vi "LD2018_ブロック崩し_Main.vi"() -> ()   [LabVIEW 2016]
uses:
  <vilib>/Utility/inputDevices.llb/keyboardAcquire.vi
  <vilib>/Utility/inputDevices.llb/closeKeyboard.vi
panel:
  out "Stage":i32
  out "残機":i32
  out "Combo":i32
  out "Combo":bool
  out "SCORE":i32
  out "BL 0":bool
  out "BL 1":bool
  out "BL 2":bool
  out "BL 3":bool
  out "BL 4":bool
  out "BL 5":bool
  out "BL 6":bool
  out "BL 7":bool
  out "BL 8":bool
  out "BL 9":bool
  out "BL 10":bool
  out "BL 11":bool
  out "BL 12":bool
  out "BL 13":bool
  out "BL 14":bool
  out "BL 15":bool
  out "BL 16":bool
  out "BL 17":bool
  out "BL 18":bool
  out "BL 19":bool
  out "BL 20":bool
  out "BL 21":bool
  out "BL 22":bool
  out "BL 23":bool
  out "BL 24":bool
  out "BL 25":bool
  out "BL 26":bool
  out "BL 27":bool
  out "BL 28":bool
  out "BL 29":bool
  out "BL 30":bool
  out "BL 31":bool
  out "BL 32":bool
  out "BL 33":bool
  out "BL 34":bool
  out "BL 35":bool
  out "BL 36":bool
  out "BL 37":bool
  out "BL 38":bool
  out "BL 39":bool
  out "BL 40":bool
  out "BL 41":bool
  out "BL 42":bool
  out "BL 43":bool
  out "BL 44":bool
  out "BL 45":bool
  out "BL 46":bool
  out "BL 47":bool
  out "BL 48":bool
  out "BL 49":bool
  out "BL 50":bool
  out "BL 51":bool
  out "BL 52":bool
  out "BL 53":bool
  out "BL 54":bool
  out "BL 55":bool
  out "BL 56":bool
  out "BL 57":bool
  out "BL 58":bool
  out "BL 59":bool
  out "BL 60":bool
  out "BL 61":bool
  out "BL 62":bool
  out "BL 63":bool
  out "BL 64":bool
  out "BL 65":bool
  out "BL 66":bool
  out "BL 67":bool
  out "BL 68":bool
  out "BL 69":bool
  out "BL 70":bool
  out "BL 71":bool
  out "BL 72":bool
  out "BL 73":bool
  out "BL 74":bool
  out "BL 75":bool
  out "BL 76":bool
  out "BL 77":bool
  out "BL 78":bool
  out "BL 79":bool
  out "BL 80":bool
  out "BL 81":bool
  out "BL 82":bool
  out "BL 83":bool
  out "BL 84":bool
  out "BL 85":bool
  out "BL 86":bool
  out "BL 87":bool
  out "BL 88":bool
  out "BL 89":bool
  out "BL 90":bool
  out "BL 91":bool
  out "BL 92":bool
  out "BL 93":bool
  out "BL 94":bool
  out "BL 95":bool
  out "BL 96":bool
  out "BL 97":bool
  out "BL 98":bool
  out "BL 99":bool
  out "BL 100":bool
  out "BL 110":bool
  out "BL 120":bool
  out "BL 130":bool
  out "BL 140":bool
  out "BL 101":bool
  out "BL 111":bool
  out "BL 121":bool
  out "BL 131":bool
  out "BL 141":bool
  out "BL 102":bool
  out "BL 112":bool
  out "BL 122":bool
  out "BL 132":bool
  out "BL 142":bool
  out "BL 103":bool
  out "BL 113":bool
  out "BL 123":bool
  out "BL 133":bool
  out "BL 143":bool
  out "BL 104":bool
  out "BL 114":bool
  out "BL 124":bool
  out "BL 134":bool
  out "BL 144":bool
  out "BL 105":bool
  out "BL 115":bool
  out "BL 125":bool
  out "BL 135":bool
  out "BL 145":bool
  out "BL 106":bool
  out "BL 116":bool
  out "BL 126":bool
  out "BL 136":bool
  out "BL 146":bool
  out "BL 107":bool
  out "BL 117":bool
  out "BL 127":bool
  out "BL 137":bool
  out "BL 147":bool
  out "BL 108":bool
  out "BL 118":bool
  out "BL 128":bool
  out "BL 138":bool
  out "BL 148":bool
  out "BL 109":bool
  out "BL 119":bool
  out "BL 129":bool
  out "BL 139":bool
  out "BL 149":bool
  out "x - y":u32
  in  "rect":T1={"left"=175, "top"=550, "right"=224, "bottom"=565} caption="長方形"
  out "Scrn-PADDLE":picture
  out "Scrn-BALL":picture
  # "BGカラーを黒(#000000)にすると\n処理速度が上がる？"
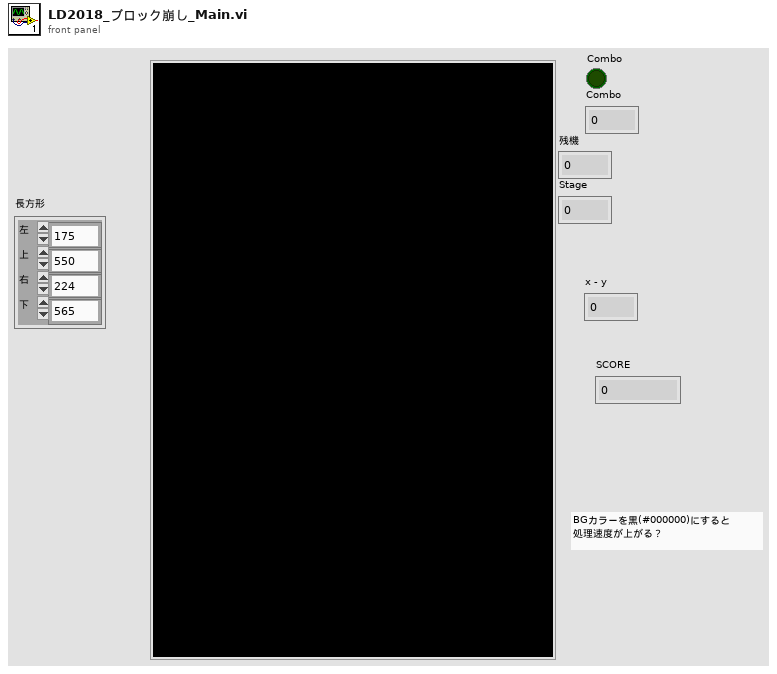
[diagram p1: front panel]
types:
  T1 = cluster{"left":i16, "top":i16, "right":i16, "bottom":i16}
  T2 = cluster{"left":dbl, "top":dbl, "right":dbl, "bottom":dbl}
  T3 = enum16{"0", "1", "2", "3", "4", "5", "6", "7", "8", "9", "A", "B", "C", "D", "E", "F", "G", "H", "I", "J", "K", "L", "M", "N", "O", "P", "Q", "R", "S", "T", "U", "V", "W", "X", "Y", "Z", "F1", "F2", "F3", "F4", "F5", "F6", "F7", "F8", "F9", "F10", "F11", "F12", "F13", "F14", "F15", "ADD", "BACK", "BACKSLASH", "CAPITAL", "COMMA", "DECIMAL", "DELETE", "DIVIDE", "DOWN", "END", "EQUALS", "ESCAPE", "GRAVE (`)", "HOME", "INSERT", "LBRACKET", "LCONTROL", "LEFT", "L ALT", "LSHIFT", "LWIN", "MINUS", "MULTIPLY", "NEXT", "NUMLOCK", "NUMPAD_0", "NUMPAD_1", "NUMPAD_2", "NUMPAD_3", "NUMPAD_4", "NUMPAD_5", "NUMPAD_6", "NUMPAD_7", "NUMPAD_8", "NUMPAD_9", "PAUSE", "PERIOD", "PRIOR (PG UP)", "RBRACKET", "RCONTROL", "RETURN", "RIGHT", "R ALT", "RSHIFT", "RWIN", "SCROLL", "SEMICOLON", "SLASH", "SPACE", "SUBTRACT", "TAB", "UP", "ENTER (num pad)", "' (quote)"}[]
  T4 = typedef "LVPositionTypeDef.ctl" = cluster{"Left":i32, "Top":i32}
  T5 = enum16{"0", "1", "2", "3", "4", "5", "6", "7", "8", "9", "A", "B", "C", "D", "E", "F", "G", "H", "I", "J", "K", "L", "M", "N", "O", "P", "Q", "R", "S", "T", "U", "V", "W", "X", "Y", "Z", "F1", "F2", "F3", "F4", "F5", "F6", "F7", "F8", "F9", "F10", "F11", "F12", "F13", "F14", "F15", "ADD", "BACK", "BACKSLASH", "CAPITAL", "COMMA", "DECIMAL", "DELETE", "DIVIDE", "DOWN", "END", "EQUALS", "ESCAPE", "GRAVE (`)", "HOME", "INSERT", "LBRACKET", "LCONTROL", "LEFT", "L ALT", "LSHIFT", "LWIN", "MINUS", "MULTIPLY", "NEXT", "NUMLOCK", "NUMPAD_0", "NUMPAD_1", "NUMPAD_2", "NUMPAD_3", "NUMPAD_4", "NUMPAD_5", "NUMPAD_6", "NUMPAD_7", "NUMPAD_8", "NUMPAD_9", "PAUSE", "PERIOD", "PRIOR (PG UP)", "RBRACKET", "RCONTROL", "RETURN", "RIGHT", "R ALT", "RSHIFT", "RWIN", "SCROLL", "SEMICOLON", "SLASH", "SPACE", "SUBTRACT", "TAB", "UP", "ENTER (num pad)", "' (quote)"}
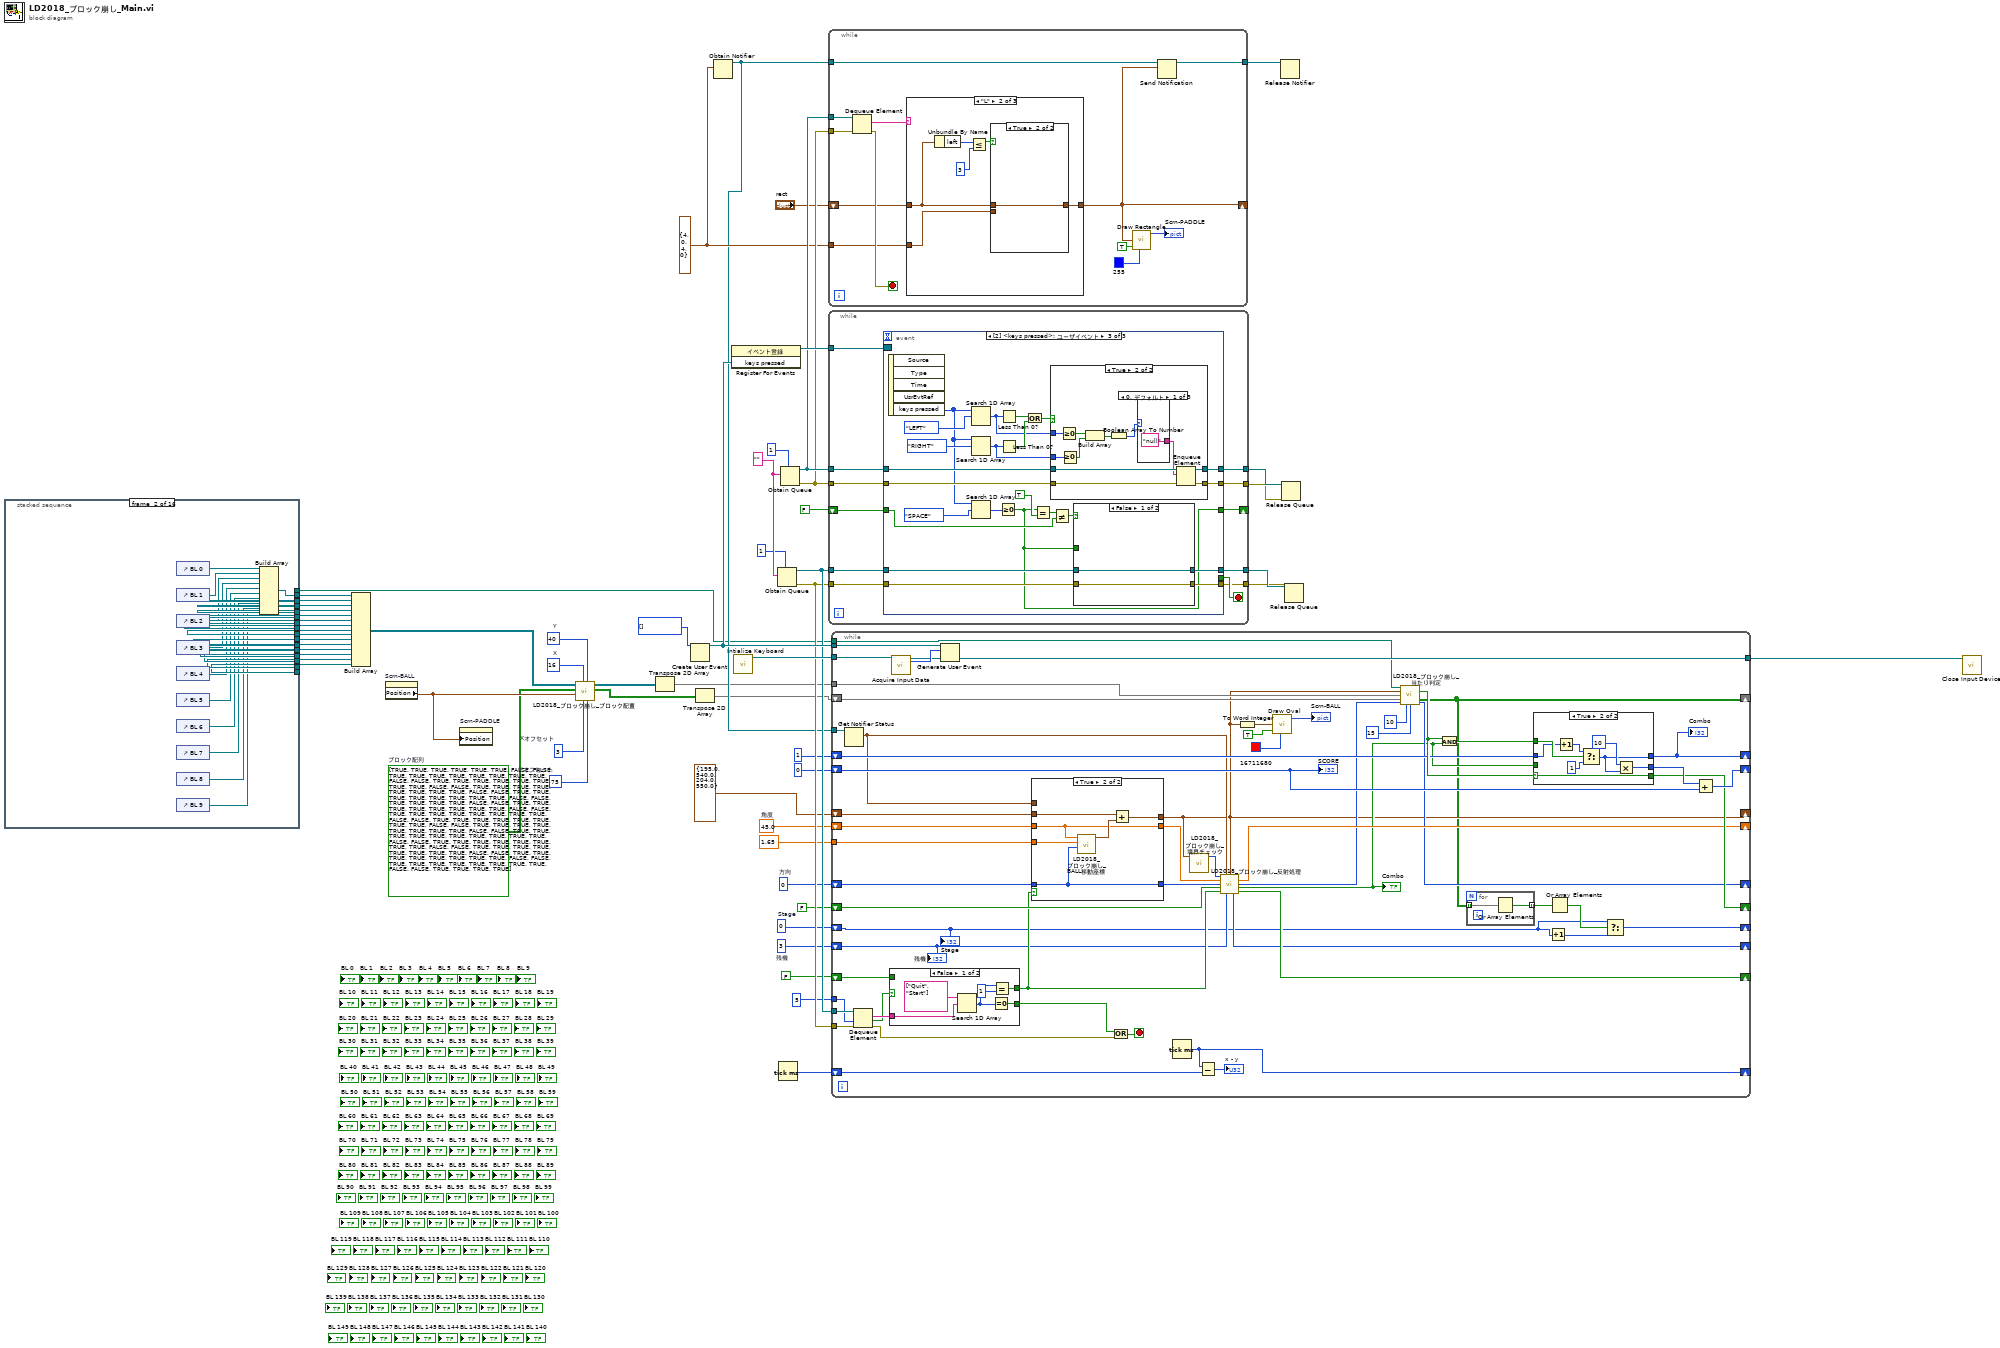
[diagram p0: block diagram]
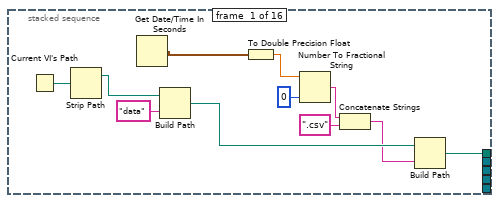
[diagram p2: hidden frame]
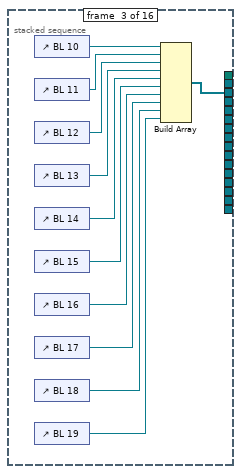
[diagram p3: hidden frame]
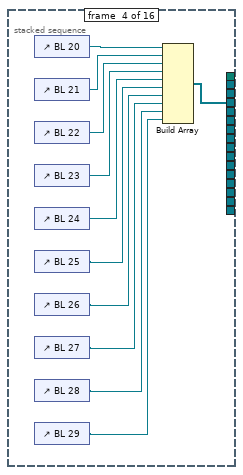
[diagram p4: hidden frame]
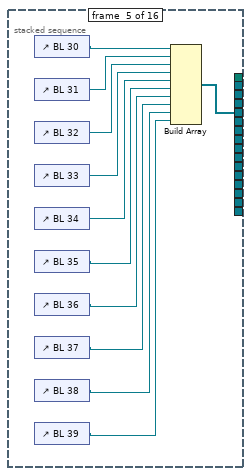
[diagram p5: hidden frame]
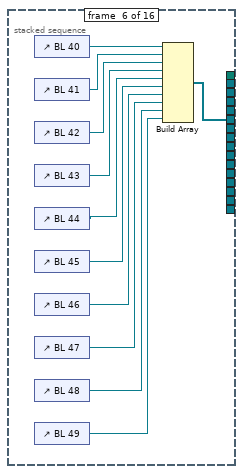
[diagram p6: hidden frame]
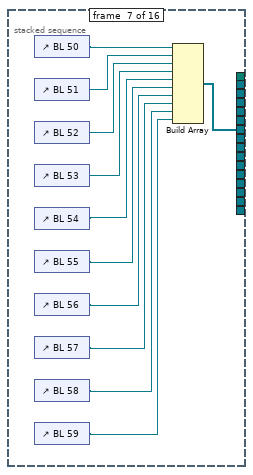
[diagram p7: hidden frame]
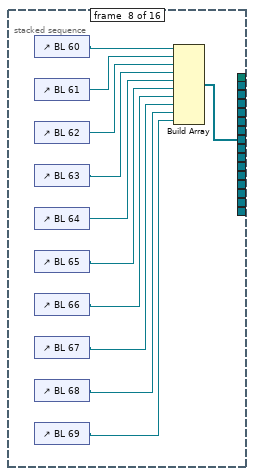
[diagram p8: hidden frame]
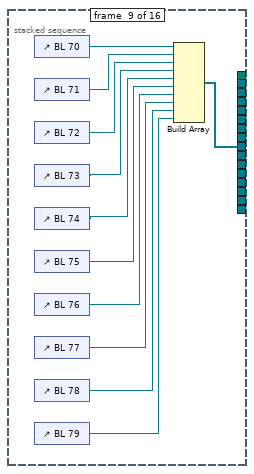
[diagram p9: hidden frame]
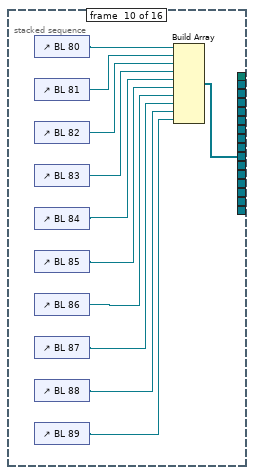
[diagram p10: hidden frame]
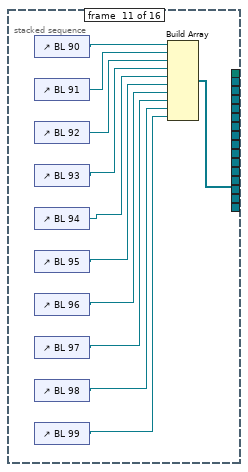
[diagram p11: hidden frame]
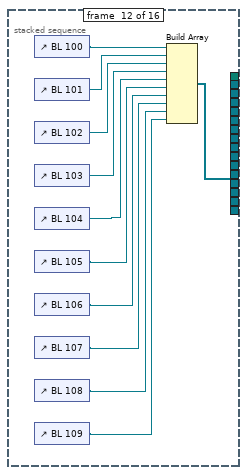
[diagram p12: hidden frame]
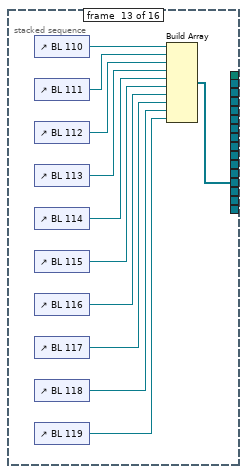
[diagram p13: hidden frame]
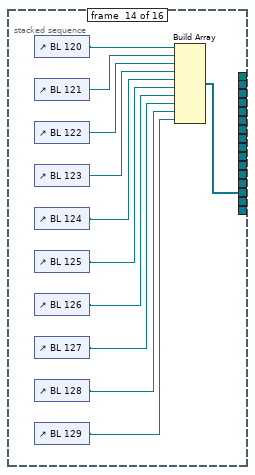
[diagram p14: hidden frame]
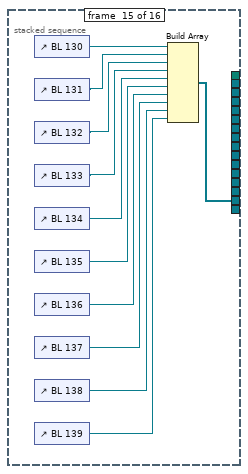
[diagram p15: hidden frame]
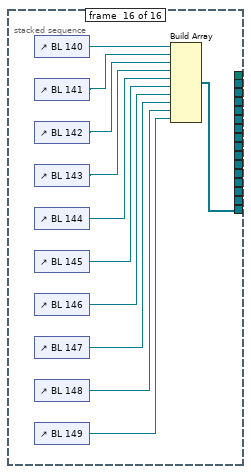
[diagram p16: hidden frame]
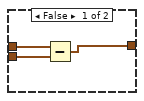
[diagram p18: hidden frame]
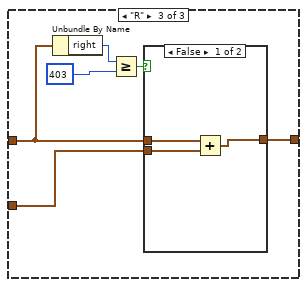
[diagram p19: hidden frame]
diagram:
  w1 = 3  # 残機
  w2 = 0  # Stage
  w8 = 75  # Yオフセット
  w9 = 3  # Xオフセット
  w10 = 40  # Y
  w11 = 16  # X
  w5 = bool[][] [[TRUE, TRUE, TRUE, TRUE, TRUE, TRUE, FALSE, FALSE, TRUE, TRUE], [TRUE, TRUE, TRUE, TRUE, TRUE, TRUE, FALSE, FALSE, TRUE, TRUE], [TRUE, TRUE, TRUE, TRUE, TRUE, TRUE, FALSE, FALSE, TRUE, TRUE], [TRUE, TRUE, TRUE, TRUE, TRUE, TRUE, FALSE, FALSE, TRUE, TRUE], [TRUE, TRUE, TRUE, TRUE, TRUE, TRUE, FALSE, FALSE, TRUE, TRUE], [TRUE, TRUE, FALSE, FALSE, TRUE, TRUE, TRUE, TRUE, TRUE, TRUE], [TRUE, TRUE, FALSE, FALSE, TRUE, TRUE, TRUE, TRUE, TRUE, TRUE], [TRUE, TRUE, FALSE, FALSE, TRUE, TRUE, TRUE, TRUE, TRUE, TRUE], [TRUE, TRUE, FALSE, FALSE, TRUE, TRUE, TRUE, TRUE, TRUE, TRUE], [TRUE, TRUE, FALSE, FALSE, TRUE, TRUE, TRUE, TRUE, TRUE, TRUE], [TRUE, TRUE, TRUE, TRUE, FALSE, FALSE, TRUE, TRUE, TRUE, TRUE], [TRUE, TRUE, TRUE, TRUE, FALSE, FALSE, TRUE, TRUE, TRUE, TRUE], [TRUE, TRUE, TRUE, TRUE, FALSE, FALSE, TRUE, TRUE, TRUE, TRUE], [TRUE, TRUE, TRUE, TRUE, FALSE, FALSE, TRUE, TRUE, TRUE, TRUE], [TRUE, TRUE, TRUE, TRUE, FALSE, FALSE, TRUE, TRUE, TRUE, TRUE]]  # ブロック配列
  w44 = 0  # 方向
  w45 = 45.0  # 角度
  w33 = T1 {"left"=4, "top"=0, "right"=4, "bottom"=0} ("rect")
  w16 = ""
  w59 = T3 [] items=["0", "1", "2", "3", "4", "5", "6", "7", "8", "9", "A", "B", "C", "D", "E", "F", "G", "H", "I", "J", "K", "L", "M", "N", "O", "P", "Q", "R", "S", "T", "U", "V", "W", "X", "Y", "Z", "F1", "F2", "F3", "F4", "F5", "F6", "F7", "F8", "F9", "F10", "F11", "F12", "F13", "F14", "F15", "ADD", "BACK", "BACKSLASH", "CAPITAL", "COMMA", "DECIMAL", "DELETE", "DIVIDE", "DOWN", "END", "EQUALS", "ESCAPE", "GRAVE (`)", "HOME", "INSERT", "LBRACKET", "LCONTROL", "LEFT", "L ALT", "LSHIFT", "LWIN", "MINUS", "MULTIPLY", "NEXT", "NUMLOCK", "NUMPAD_0", "NUMPAD_1", "NUMPAD_2", "NUMPAD_3", "NUMPAD_4", "NUMPAD_5", "NUMPAD_6", "NUMPAD_7", "NUMPAD_8", "NUMPAD_9", "PAUSE", "PERIOD", "PRIOR (PG UP)", "RBRACKET", "RCONTROL", "RETURN", "RIGHT", "R ALT", "RSHIFT", "RWIN", "SCROLL", "SEMICOLON", "SLASH", "SPACE", "SUBTRACT", "TAB", "UP", "ENTER (num pad)", "' (quote)"] ("keys pressed")
  n1 = stacked-sequence {
    tunnel: [_ w72 _ _ _ _ _ _ _ _ _ _ _ _ _ _] -> w43
    tunnel: [_ _ w83 _ _ _ _ _ _ _ _ _ _ _ _ _] -> w42
    tunnel: [_ _ _ w104 _ _ _ _ _ _ _ _ _ _ _ _] -> w41
    tunnel: [_ _ _ _ w115 _ _ _ _ _ _ _ _ _ _ _] -> w40
    tunnel: [_ _ _ _ _ w126 _ _ _ _ _ _ _ _ _ _] -> w39
    tunnel: [_ _ _ _ _ _ w137 _ _ _ _ _ _ _ _ _] -> w38
    tunnel: [_ _ _ _ _ _ _ w148 _ _ _ _ _ _ _ _] -> w37
    tunnel: [_ _ _ _ _ _ _ _ w159 _ _ _ _ _ _ _] -> w36
    tunnel: [_ _ _ _ _ _ _ _ _ w170 _ _ _ _ _ _] -> w35
    tunnel: [_ _ _ _ _ _ _ _ _ _ w181 _ _ _ _ _] -> w34
    tunnel: [_ _ _ _ _ _ _ _ _ _ _ w182 _ _ _ _] -> w27
    tunnel: [_ _ _ _ _ _ _ _ _ _ _ _ w193 _ _ _] -> w26
    tunnel: [_ _ _ _ _ _ _ _ _ _ _ _ _ w205 _ _] -> w25
    tunnel: [_ _ _ _ _ _ _ _ _ _ _ _ _ _ w215 _] -> w24
    tunnel: [_ _ _ _ _ _ _ _ _ _ _ _ _ _ _ w226] -> w23
    tunnel: [w62 _ _ _ _ _ _ _ _ _ _ _ _ _ _ _] -> w20
    frame #0 {
      n2 = Current VI's Path() -> (path=w69:path)
      n3 = Strip Path(path=w69) -> (stripped path=w70:path)  [unwired: 1 out]
      n4 = Get Date/Time In Seconds() -> (seconds since 1Jan1904=w61:timestamp)
      n5 = Build Path(base path=w70, name or relative path="data" ("名前または相対パス")) -> (appended path=w64:path)
      n6 = To Double Precision Float(number=w61) -> (double precision float=w68:dbl)
      n7 = Number To Fractional String(number=w68, precision (6)=i16 0 ("精度（6）")) -> (F-format string=w66:string)  [unwired: 2 in]
      n8 = Concatenate Strings(w66, ".csv" ("文字列")) -> (w63:string)
      n9 = Build Path(base path=w64, name or relative path=w63) -> (appended path=w62:path)
    }
    frame #1 {
      n10 = control-ref of="BL 0"() -> (w73:refnum<vi>)
      n11 = control-ref of="BL 1"() -> (w74:refnum<vi>)
      n12 = control-ref of="BL 2"() -> (w75:refnum<vi>)
      n13 = control-ref of="BL 3"() -> (w76:refnum<vi>)
      n14 = control-ref of="BL 4"() -> (w77:refnum<vi>)
      n15 = control-ref of="BL 5"() -> (w78:refnum<vi>)
      n16 = control-ref of="BL 6"() -> (w79:refnum<vi>)
      n17 = control-ref of="BL 7"() -> (w80:refnum<vi>)
      n18 = control-ref of="BL 8"() -> (w81:refnum<vi>)
      n19 = control-ref of="BL 9"() -> (w82:refnum<vi>)
      n20 = Build Array(w73, w74, w75, w76, w77, w78, w79, w80, w81, w82) -> (w72:refnum<vi>[])
    }
    frame #2 {
      n21 = control-ref of="BL 10"() -> (w93:refnum<vi>)
      n22 = control-ref of="BL 11"() -> (w92:refnum<vi>)
      n23 = control-ref of="BL 12"() -> (w91:refnum<vi>)
      n24 = control-ref of="BL 13"() -> (w90:refnum<vi>)
      n25 = control-ref of="BL 14"() -> (w89:refnum<vi>)
      n26 = control-ref of="BL 15"() -> (w88:refnum<vi>)
      n27 = control-ref of="BL 16"() -> (w87:refnum<vi>)
      n28 = control-ref of="BL 17"() -> (w86:refnum<vi>)
      n29 = control-ref of="BL 18"() -> (w85:refnum<vi>)
      n30 = control-ref of="BL 19"() -> (w84:refnum<vi>)
      n31 = Build Array(w93, w92, w91, w90, w89, w88, w87, w86, w85, w84) -> (w83:refnum<vi>[])
    }
    frame #3 {
      n32 = control-ref of="BL 20"() -> (w103:refnum<vi>)
      n33 = control-ref of="BL 21"() -> (w102:refnum<vi>)
      n34 = control-ref of="BL 22"() -> (w101:refnum<vi>)
      n35 = control-ref of="BL 23"() -> (w100:refnum<vi>)
      n36 = control-ref of="BL 24"() -> (w99:refnum<vi>)
      n37 = control-ref of="BL 25"() -> (w98:refnum<vi>)
      n38 = control-ref of="BL 26"() -> (w97:refnum<vi>)
      n39 = control-ref of="BL 27"() -> (w96:refnum<vi>)
      n40 = control-ref of="BL 28"() -> (w95:refnum<vi>)
      n41 = control-ref of="BL 29"() -> (w94:refnum<vi>)
      n42 = Build Array(w103, w102, w101, w100, w99, w98, w97, w96, w95, w94) -> (w104:refnum<vi>[])
    }
    frame #4 {
      n43 = control-ref of="BL 30"() -> (w114:refnum<vi>)
      n44 = control-ref of="BL 31"() -> (w113:refnum<vi>)
      n45 = control-ref of="BL 32"() -> (w112:refnum<vi>)
      n46 = control-ref of="BL 33"() -> (w111:refnum<vi>)
      n47 = control-ref of="BL 34"() -> (w110:refnum<vi>)
      n48 = control-ref of="BL 35"() -> (w109:refnum<vi>)
      n49 = control-ref of="BL 36"() -> (w108:refnum<vi>)
      n50 = control-ref of="BL 37"() -> (w107:refnum<vi>)
      n51 = control-ref of="BL 38"() -> (w106:refnum<vi>)
      n52 = control-ref of="BL 39"() -> (w105:refnum<vi>)
      n53 = Build Array(w114, w113, w112, w111, w110, w109, w108, w107, w106, w105) -> (w115:refnum<vi>[])
    }
    frame #5 {
      n54 = control-ref of="BL 40"() -> (w125:refnum<vi>)
      n55 = control-ref of="BL 41"() -> (w124:refnum<vi>)
      n56 = control-ref of="BL 42"() -> (w123:refnum<vi>)
      n57 = control-ref of="BL 43"() -> (w122:refnum<vi>)
      n58 = control-ref of="BL 44"() -> (w121:refnum<vi>)
      n59 = control-ref of="BL 45"() -> (w120:refnum<vi>)
      n60 = control-ref of="BL 46"() -> (w119:refnum<vi>)
      n61 = control-ref of="BL 47"() -> (w118:refnum<vi>)
      n62 = control-ref of="BL 48"() -> (w117:refnum<vi>)
      n63 = control-ref of="BL 49"() -> (w116:refnum<vi>)
      n64 = Build Array(w125, w124, w123, w122, w121, w120, w119, w118, w117, w116) -> (w126:refnum<vi>[])
    }
    frame #6 {
      n65 = control-ref of="BL 50"() -> (w136:refnum<vi>)
      n66 = control-ref of="BL 51"() -> (w135:refnum<vi>)
      n67 = control-ref of="BL 52"() -> (w134:refnum<vi>)
      n68 = control-ref of="BL 53"() -> (w133:refnum<vi>)
      n69 = control-ref of="BL 54"() -> (w132:refnum<vi>)
      n70 = control-ref of="BL 55"() -> (w131:refnum<vi>)
      n71 = control-ref of="BL 56"() -> (w130:refnum<vi>)
      n72 = control-ref of="BL 57"() -> (w129:refnum<vi>)
      n73 = control-ref of="BL 58"() -> (w128:refnum<vi>)
      n74 = control-ref of="BL 59"() -> (w127:refnum<vi>)
      n75 = Build Array(w136, w135, w134, w133, w132, w131, w130, w129, w128, w127) -> (w137:refnum<vi>[])
    }
    frame #7 {
      n76 = control-ref of="BL 60"() -> (w147:refnum<vi>)
      n77 = control-ref of="BL 61"() -> (w146:refnum<vi>)
      n78 = control-ref of="BL 62"() -> (w145:refnum<vi>)
      n79 = control-ref of="BL 63"() -> (w144:refnum<vi>)
      n80 = control-ref of="BL 64"() -> (w143:refnum<vi>)
      n81 = control-ref of="BL 65"() -> (w142:refnum<vi>)
      n82 = control-ref of="BL 66"() -> (w141:refnum<vi>)
      n83 = control-ref of="BL 67"() -> (w140:refnum<vi>)
      n84 = control-ref of="BL 68"() -> (w139:refnum<vi>)
      n85 = control-ref of="BL 69"() -> (w138:refnum<vi>)
      n86 = Build Array(w147, w146, w145, w144, w143, w142, w141, w140, w139, w138) -> (w148:refnum<vi>[])
    }
    frame #8 {
      n87 = control-ref of="BL 70"() -> (w158:refnum<vi>)
      n88 = control-ref of="BL 71"() -> (w157:refnum<vi>)
      n89 = control-ref of="BL 72"() -> (w156:refnum<vi>)
      n90 = control-ref of="BL 73"() -> (w155:refnum<vi>)
      n91 = control-ref of="BL 74"() -> (w154:refnum<vi>)
      n92 = control-ref of="BL 75"() -> (w153:refnum<vi>)
      n93 = control-ref of="BL 76"() -> (w152:refnum<vi>)
      n94 = control-ref of="BL 77"() -> (w151:refnum<vi>)
      n95 = control-ref of="BL 78"() -> (w150:refnum<vi>)
      n96 = control-ref of="BL 79"() -> (w149:refnum<vi>)
      n97 = Build Array(w158, w157, w156, w155, w154, w153, w152, w151, w150, w149) -> (w159:refnum<vi>[])
    }
    frame #9 {
      n98 = control-ref of="BL 80"() -> (w169:refnum<vi>)
      n99 = control-ref of="BL 81"() -> (w168:refnum<vi>)
      n100 = control-ref of="BL 82"() -> (w167:refnum<vi>)
      n101 = control-ref of="BL 83"() -> (w166:refnum<vi>)
      n102 = control-ref of="BL 84"() -> (w165:refnum<vi>)
      n103 = control-ref of="BL 85"() -> (w164:refnum<vi>)
      n104 = control-ref of="BL 86"() -> (w163:refnum<vi>)
      n105 = control-ref of="BL 87"() -> (w162:refnum<vi>)
      n106 = control-ref of="BL 88"() -> (w161:refnum<vi>)
      n107 = control-ref of="BL 89"() -> (w160:refnum<vi>)
      n108 = Build Array(w169, w168, w167, w166, w165, w164, w163, w162, w161, w160) -> (w170:refnum<vi>[])
    }
    frame #10 {
      n109 = control-ref of="BL 90"() -> (w180:refnum<vi>)
      n110 = control-ref of="BL 91"() -> (w179:refnum<vi>)
      n111 = control-ref of="BL 92"() -> (w178:refnum<vi>)
      n112 = control-ref of="BL 93"() -> (w177:refnum<vi>)
      n113 = control-ref of="BL 94"() -> (w176:refnum<vi>)
      n114 = control-ref of="BL 95"() -> (w175:refnum<vi>)
      n115 = control-ref of="BL 96"() -> (w174:refnum<vi>)
      n116 = control-ref of="BL 97"() -> (w173:refnum<vi>)
      n117 = control-ref of="BL 98"() -> (w172:refnum<vi>)
      n118 = control-ref of="BL 99"() -> (w171:refnum<vi>)
      n119 = Build Array(w180, w179, w178, w177, w176, w175, w174, w173, w172, w171) -> (w181:refnum<vi>[])
    }
    frame #11 {
      n120 = control-ref of="BL 100"() -> (w192:refnum<vi>)
      n121 = control-ref of="BL 101"() -> (w191:refnum<vi>)
      n122 = control-ref of="BL 102"() -> (w190:refnum<vi>)
      n123 = control-ref of="BL 103"() -> (w189:refnum<vi>)
      n124 = control-ref of="BL 104"() -> (w188:refnum<vi>)
      n125 = control-ref of="BL 105"() -> (w187:refnum<vi>)
      n126 = control-ref of="BL 106"() -> (w186:refnum<vi>)
      n127 = control-ref of="BL 107"() -> (w185:refnum<vi>)
      n128 = control-ref of="BL 108"() -> (w184:refnum<vi>)
      n129 = control-ref of="BL 109"() -> (w183:refnum<vi>)
      n130 = Build Array(w192, w191, w190, w189, w188, w187, w186, w185, w184, w183) -> (w182:refnum<vi>[])
    }
    frame #12 {
      n131 = control-ref of="BL 110"() -> (w203:refnum<vi>)
      n132 = control-ref of="BL 111"() -> (w202:refnum<vi>)
      n133 = control-ref of="BL 112"() -> (w201:refnum<vi>)
      n134 = control-ref of="BL 113"() -> (w200:refnum<vi>)
      n135 = control-ref of="BL 114"() -> (w199:refnum<vi>)
      n136 = control-ref of="BL 115"() -> (w198:refnum<vi>)
      n137 = control-ref of="BL 116"() -> (w197:refnum<vi>)
      n138 = control-ref of="BL 117"() -> (w196:refnum<vi>)
      n139 = control-ref of="BL 118"() -> (w195:refnum<vi>)
      n140 = control-ref of="BL 119"() -> (w194:refnum<vi>)
      n141 = Build Array(w203, w202, w201, w200, w199, w198, w197, w196, w195, w194) -> (w193:refnum<vi>[])
    }
    frame #13 {
      n142 = control-ref of="BL 120"() -> (w214:refnum<vi>)
      n143 = control-ref of="BL 121"() -> (w213:refnum<vi>)
      n144 = control-ref of="BL 122"() -> (w212:refnum<vi>)
      n145 = control-ref of="BL 123"() -> (w211:refnum<vi>)
      n146 = control-ref of="BL 124"() -> (w210:refnum<vi>)
      n147 = control-ref of="BL 125"() -> (w209:refnum<vi>)
      n148 = control-ref of="BL 126"() -> (w204:refnum<vi>)
      n149 = control-ref of="BL 127"() -> (w208:refnum<vi>)
      n150 = control-ref of="BL 128"() -> (w207:refnum<vi>)
      n151 = control-ref of="BL 129"() -> (w206:refnum<vi>)
      n152 = Build Array(w214, w213, w212, w211, w210, w209, w204, w208, w207, w206) -> (w205:refnum<vi>[])
    }
    frame #14 {
      n153 = control-ref of="BL 130"() -> (w225:refnum<vi>)
      n154 = control-ref of="BL 131"() -> (w224:refnum<vi>)
      n155 = control-ref of="BL 132"() -> (w223:refnum<vi>)
      n156 = control-ref of="BL 133"() -> (w222:refnum<vi>)
      n157 = control-ref of="BL 134"() -> (w221:refnum<vi>)
      n158 = control-ref of="BL 135"() -> (w220:refnum<vi>)
      n159 = control-ref of="BL 136"() -> (w219:refnum<vi>)
      n160 = control-ref of="BL 137"() -> (w218:refnum<vi>)
      n161 = control-ref of="BL 138"() -> (w217:refnum<vi>)
      n162 = control-ref of="BL 139"() -> (w216:refnum<vi>)
      n163 = Build Array(w225, w224, w223, w222, w221, w220, w219, w218, w217, w216) -> (w215:refnum<vi>[])
    }
    frame #15 {
      n164 = control-ref of="BL 140"() -> (w236:refnum<vi>)
      n165 = control-ref of="BL 141"() -> (w235:refnum<vi>)
      n166 = control-ref of="BL 142"() -> (w234:refnum<vi>)
      n167 = control-ref of="BL 143"() -> (w233:refnum<vi>)
      n168 = control-ref of="BL 144"() -> (w232:refnum<vi>)
      n169 = control-ref of="BL 145"() -> (w231:refnum<vi>)
      n170 = control-ref of="BL 146"() -> (w230:refnum<vi>)
      n171 = control-ref of="BL 147"() -> (w229:refnum<vi>)
      n172 = control-ref of="BL 148"() -> (w228:refnum<vi>)
      n173 = control-ref of="BL 149"() -> (w227:refnum<vi>)
      n174 = Build Array(w236, w235, w234, w233, w232, w231, w230, w229, w228, w227) -> (w226:refnum<vi>[])
    }
  }
  n175 = Build Array(w43, w42, w41, w40, w39, w38, w37, w36, w35, w34, w27, w26, w25, w24, w23) -> (w7:refnum<vi>[][])
  n176 = property on="Scrn-BALL" class="Pict"() -> ("Position"=w6:T4)  [unwired: 2 in, 2 out]
  n177 = property on="Scrn-PADDLE" class="Pict"("Position"=w6) -> ()  [unwired: 2 in, 2 out]
  n178 = call "LD2018_ブロック崩し_ブロック配置.vi"("Yオフセット"=w8, "Y"=w10, "Xオフセット"=w9, "X"=w11, "Scrn-BALL位置"=w6, "ブロック配列入力"=w5, "ブッロクReference"=w7) -> ("ブロック配列出力"=w3:bool[][], "ブッロクReference出力"=w4:refnum<vi>[][])  [unwired: 3 in]
  n179 = Transpose 2D Array(2D array=w4) -> (transposed array=w30:refnum<vi>[][])
  n180 = Create User Event(user event datatype=w59) -> (user event=w60:refnum<user-event>)  [unwired: 1 in, 1 out]
  n181 = Transpose 2D Array(2D array=w3) -> (transposed array=w29:bool[][])
  n182 = Obtain Notifier(notification data type=w33) -> (notifier out=w31:refnum<notifier>)  [unwired: 3 in, 2 out]
  n183 = register-events(w60) -> (reference out=w56:refnum<event-registration>)  [unwired: 2 in, 1 out]
  n184 = call <vilib>:"Intialize Keyboard.vi"() -> ("device ID"=w58:refnum<k1>)  [unwired: 10 in, 1 out]
  n185 = Obtain Queue(max queue size (-1, unlimited)=1 ("最大キューサイズ（-1, 無制限）"), element data type=w16) -> (queue out=w53:refnum<queue>, error out=w52:errorcluster)  [unwired: 3 in, 1 out]
  n186 = Tick Count (ms)() -> (millisecond timer value=w28:u32)
  n187 = Obtain Queue(max queue size (-1, unlimited)=1 ("最大キューサイズ（-1, 無制限）"), element data type=w16) -> (queue out=w48:refnum<queue>, error out=w47:errorcluster)  [unwired: 3 in, 1 out]
  n188 = while {
    tunnel: w56 -> [w248]
    tunnel: w53 -> [w246]
    tunnel: w52 -> [w245]
    tunnel: [w244] -> w55
    tunnel: [w243] -> w54
    tunnel: w48 -> [w242]
    tunnel: w47 -> [w241]
    tunnel: [w240] -> w51
    tunnel: [w239] -> w50
    shift-right: [w237] -> _
    shift-left: FALSE -> [w238]
    stop <- w247 stop-if-true
    n189 = event shown="[2] <keys pressed>: ユーザイベント" {
      selector: w248 -> [_ _ _]
      dyn-events: _ -> [_ _ _]
      timeout: _ -> [_ _ _]
      tunnel: [_ w262 _] -> w247
      tunnel: w246 -> [w251 w261 w271]
      tunnel: w245 -> [w250 w260 w270]
      tunnel: [w251 w259 w269] -> w244
      tunnel: [w250 w258 w268] -> w243
      tunnel: w242 -> [w253 w257 w285]
      tunnel: w241 -> [w252 w256 w284]
      tunnel: [w253 w257 w276] -> w240
      tunnel: [w252 w256 w275] -> w239
      tunnel: w238 -> [w249 w254 w265]
      tunnel: [w249 w254 w263] -> w237
      event Timeout {
        n190 = event-data() -> ()  [unwired: 1 in, 2 out]
      }
      event Panel Close? {
        (unwired) "Quit" ("要素")
        w262 = TRUE ("破棄?")
        n191 = event-data() -> ()  [unwired: 1 in, 4 out]
        n192 = Enqueue Element(queue=w261, element="Quit" ("要素"), error in (no error)=w260) -> (queue out=w259:refnum<queue>, error out=w258:errorcluster)  [unwired: 1 in, 1 out]
        n193 = event-data("Discard?"=w262) -> ()  [unwired: 1 in, 1 out]
      }
      event User Event {
        n194 = event-data() -> ("keys pressed"=w274:T3)  [unwired: 1 in, 4 out]
        n195 = Search 1D Array(1D array=w274, element=T5."RIGHT" ("要素")) -> (index of element=w277:i32)  [unwired: 1 in]
        n196 = Search 1D Array(1D array=w274, element=T5."LEFT" ("要素")) -> (index of element=w278:i32)  [unwired: 1 in]
        n197 = Search 1D Array(1D array=w274, element=T5."SPACE" ("要素")) -> (index of element=w272:i32)  [unwired: 1 in]
        n198 = Greater Or Equal To 0?(x=w272) -> (x >= 0?=w263:bool)
        n199 = Less Than 0?(x=w278) -> (x < 0?=w281:bool)
        n200 = Less Than 0?(x=w277) -> (x < 0?=w280:bool)
        n201 = Or(x=w281, y=w280) -> (x .or. y?=w279:bool)
        n202 = Equal?(x=w263, y=TRUE) -> (x = y?=w266:bool)
        n203 = case shown="TRUE" w279 {
          tunnel: w285 -> [w301 w312]
          tunnel: w284 -> [w300 w311]
          tunnel: w278 -> [_ w308]
          tunnel: w277 -> [_ w307]
          tunnel: [w301 w310] -> w276
          tunnel: [w300 w309] -> w275
          frame False {
          }
          frame True {
            n204 = Greater Or Equal To 0?(x=w308) -> (x >= 0?=w306:bool)
            n205 = Greater Or Equal To 0?(x=w307) -> (x >= 0?=w305:bool)
            n206 = Build Array(w306, w305) -> (w304:bool[])
            n207 = Boolean Array To Number(Boolean array=w304) -> (number=w303:u32)
            n208 = case shown="0, デフォルト" w303 {
              tunnel: ["null" "L" "R"] -> w302
              frame 0, Default {
              }
              frame 1 {
              }
              frame 2 {
              }
            }
            n209 = Enqueue Element(queue=w312, element=w302, error in (no error)=w311) -> (queue out=w310:refnum<queue>, error out=w309:errorcluster)  [unwired: 1 in, 1 out]
          }
        }
        n210 = Not Equal?(x=w266, y=w265) -> (x != y?=w264:bool)
        n211 = case shown="FALSE" w264 {
          tunnel: w271 -> [w287 w292]
          tunnel: w270 -> [w286 w291]
          tunnel: [w287 w290] -> w269
          tunnel: [w286 w289] -> w268
          tunnel: w263 -> [_ w288]
          frame False {
          }
          frame True {
            n212 = case shown="TRUE" w288 {
              tunnel: w292 -> [w294 w299]
              tunnel: w291 -> [w293 w298]
              tunnel: [w294 w297] -> w290
              tunnel: [w293 w296] -> w289
              frame False {
              }
              frame True {
                n213 = Enqueue Element(queue=w299, element="Start" ("要素"), error in (no error)=w298) -> (queue out=w297:refnum<queue>, error out=w296:errorcluster)  [unwired: 1 in, 1 out]
              }
            }
          }
        }
      }
    }
  }
  n214 = while {
    tunnel: w48 -> [w327]
    tunnel: w47 -> [w326]
    shift-right: [w318] -> _
    shift-left: "rect" -> [w323]
    tunnel: w33 -> [w320]
    tunnel: w31 -> [w319]
    tunnel: [w317] -> w32
    stop <- w324 stop-if-true
    n215 = Dequeue Element(queue=w327, error in (no error)=w326) -> (element=w325:string, error out=w324:errorcluster)  [unwired: 1 in, 2 out]
    n216 = case shown="\"L\"" w325 {
      tunnel: w323 -> [w328 w333 w344]
      tunnel: [w328 w334 w343] -> w318
      tunnel: w320 -> [_ w332 w339]
      frame "null", Default {
      }
      frame "L" {
        n217 = Unbundle By Name(w333) -> ("left"=w331:i16)
        n218 = Less Or Equal?(x=w331, y=i16 3) -> (x <= y?=w329:bool)
        n219 = case shown="TRUE" w329 {
          tunnel: [w335 w338] -> w334
          tunnel: w333 -> [w337 w338]
          tunnel: w332 -> [w336 _]
          frame False {
            n220 = Subtract(x=w337, y=w336) -> (x-y=w335:T1)
          }
          frame True {
          }
        }
      }
      frame "R" {
        n221 = Unbundle By Name(w344) -> ("right"=w342:i16)
        n222 = Greater Or Equal?(x=w342, y=i16 403) -> (x >= y?=w340:bool)
        n223 = case shown="FALSE" w340 {
          tunnel: w344 -> [w347 w348]
          tunnel: [w345 w348] -> w343
          tunnel: w339 -> [w346 _]
          frame False {
            n224 = Add(x=w347, y=w346) -> (x+y=w345:T1)
          }
          frame True {
          }
        }
      }
    }
    n225 = call <vilib>:"Draw Rectangle.vi"("rect"=w318, "fill?(F)"=TRUE, "color(black)"=u32 255) -> ("new picture"=→"Scrn-PADDLE":picture)  [unwired: 6 in]
    n226 = Send Notification(notification=w318, notifier=w319) -> (notifier out=w317:refnum<notifier>)  [unwired: 1 in, 1 out]
  }
  n227 = while {
    tunnel: w60 -> [w406]
    tunnel: w58 -> [w405]
    tunnel: [w403] -> w57
    tunnel: w53 -> [w402]
    tunnel: w52 -> [w401]
    shift-right: [w359] -> _
    shift-left: T2 {"left"=195.0, "top"=540.0, "right"=204.0, "bottom"=550.0} ("rect 3") -> [w398]
    shift-right: [w365] -> _
    shift-left: w45 -> [w395]
    shift-right: [w364] -> _
    shift-left: w44 -> [w397]
    tunnel: w31 -> [w396]
    tunnel: w30 -> [w361]
    shift-right: [w354] -> _
    shift-left: w29 -> [w360]
    shift-right: [w393] -> _
    shift-left: w28 -> [w394]
    tunnel: 5 ("タイムアウト（ms）（-1）") -> [w389]
    tunnel: 1.65 -> [w388]
    tunnel: w20 -> [w377]
    shift-right: [w379] -> _
    shift-left: FALSE -> [w367]
    shift-right: [w383] -> _
    shift-left: 1 -> [w378]
    shift-right: [w381] -> _
    shift-left: 0 -> [w380]
    shift-right: [w366] -> _
    shift-left: FALSE -> [w371]
    shift-right: [w349] -> _
    shift-left: w2 -> [w351]
    shift-right: [w355] -> _
    shift-left: w1 -> [w356]
    stop <- w390 stop-if-true
    n228 = Get Notifier Status(notifier=w396) -> (current notification=w376:T1)  [unwired: 1 in, 4 out]
    n229 = Dequeue Element(queue=w402, timeout in ms (-1)=w389, error in (no error)=w401) -> (element=w375:string, timed out?=w373:bool, error out=w391:errorcluster)  [unwired: 1 out]
    n230 = case shown="FALSE" w373 {
      tunnel: w375 -> [w413 _]
      tunnel: [w412 FALSE] -> w372
      tunnel: [w409 w415] -> w357
      tunnel: w371 -> [_ w415]
      frame False {
        n231 = Search 1D Array(1D array=string[] ["Quit", "Start"], element=w413) -> (index of element=w411:i32)  [unwired: 1 in]
        n232 = Equal To 0?(x=w411) -> (x = 0?=w412:bool)
        n233 = Equal?(x=w411, y=1) -> (x = y?=w409:bool)
      }
      frame True {
      }
    }
    n234 = call-poly <vilib>:"Acquire Input Data.vi"("device ID"=w405) -> ("device ID"=w403:refnum<k1>, "keys pressed"=w404:T3)  [unwired: 16 in, 1 out]
    n235 = Generate User Event(user event=w406, event data cluster=w404) -> ()  [unwired: 2 in, 2 out]
    n236 = case shown="TRUE" w357 {
      tunnel: w398 -> [_ w433]
      tunnel: w397 -> [_ w428]
      tunnel: w395 -> [_ w429]
      tunnel: [w417 w431] -> w359
      tunnel: w388 -> [_ w430]
      tunnel: [45.0 ("角度") w429] -> w370
      tunnel: [0 ("方向") w428] -> w368
      tunnel: w376 -> [w426 _]
      frame False {
        n237 = Unbundle By Name(w426) -> ("left"=w425:i16)
        n238 = Add(x=w425, y=i16 20) -> (x+y=w421:i16)
        n239 = Add(x=w425, y=i16 30) -> (x+y=w419:i16)
        n240 = Bundle(w421, "top"=540.0, w419, "top"=550.0) -> (w417:cluster{i16, "top":dbl, i16, "top":dbl})  [unwired: 1 in]
      }
      frame True {
        n241 = call "LD2018_ブロック崩し_BALL移動座標.vi"("方向"=w428, "移動速度"=w430, "角度"=w429) -> ("座標"=w432:cluster{dbl, dbl, dbl, dbl})  [unwired: 8 in]
        n242 = Add(x=w433, y=w432) -> (x+y=w431:cluster{dbl, dbl, dbl, dbl})
      }
    }
    n243 = Or(x=w372, y=w391) -> (x .or. y?=w390:bool)
    n244 = Tick Count (ms)() -> (millisecond timer value=w393:u32)
    n245 = call "LD2018_ブロック崩し_境界チェック.vi"("Ball座標"=w359) -> ("接触点"=w369:i32)  [unwired: 10 in]
    n246 = Subtract(x=w393, y=w394) -> (x-y=→"x - y":u32)
    n247 = call "LD2018_ブロック崩し_反射処理.vi"("接触点"=w369, "PADDLE座標"=w376, "Ball座標"=w359, "角度入力"=w370, "方向入力"=w368, "Combo中入力"=w367, "Play中入力"=w357, "残機入力"=w356) -> ("角度出力"=w365:dbl, "方向出力"=w363:i32, "Combo中出力"=w362:bool, "残機出力"=w355:i32, "Play中出力"=w366:bool)  [unwired: 3 in]
    "Combo" <- w362
    n248 = To Word Integer(number=w359) -> (16bit integer=w358:cluster{i16, "top":i16, i16, "top":i16})
    n249 = call <vilib>:"Draw Oval.vi"("rect"=w358, "fill?(F)"=TRUE, "color(black)"=u32 16711680) -> ("new picture"=→"Scrn-BALL":picture)  [unwired: 6 in]
    n250 = call "LD2018_ブロック崩し_当たり判定.vi"("file path (dialog if empty)"=w377, "Ball座標"=w359, "ブロックReferences"=w361, "ブロック配列in"=w360, "方向in"=w363, "行"=10, "列"=15) -> ("Hit?"=w385:bool, "ブロック配列"=w354:bool[][], "方向out"=w364:i32)  [unwired: 6 in]
    n251 = And(x=w385, y=w362) -> (x .and. y?=w384:bool)
    n252 = for {
      tunnel: w354 -> [w408] mode=indexing
      tunnel: [w407] -> w353 mode=indexing
      n253 = Or Array Elements(Boolean array=w408) -> (logical OR=w407:bool)
    }
    n254 = case shown="TRUE" w385 {
      selector: w385 -> [_ w442]
      tunnel: w384 -> [_ w441]
      tunnel: w378 -> [w435 w440]
      tunnel: [w435 w437] -> w383
      tunnel: [0 w443] -> w382
      tunnel: [w434 w442] -> w379
      tunnel: w362 -> [w434 _]
      frame False {
      }
      frame True {
        n255 = Increment(x=w440) -> (x+1=w439:i32)
        n256 = Select(t=w439, s=w441, f=1) -> (s? t:f=w437:i32)
        n257 = Multiply(x=10, y=w437) -> (x*y=w443:i32)
      }
    }
    "Combo" <- w383
    n258 = Increment(x=w351) -> (x+1=w350:i32)
    n259 = Or Array Elements(Boolean array=w353) -> (logical OR=w352:bool)
    n260 = Select(t=w351, s=w352, f=w350) -> (s? t:f=w349:i32)
    n261 = Add(x=w382, y=w380) -> (x+y=w381:i32)
    "SCORE" <- w380
    "残機" <- w356
    "Stage" <- w351
  }
  n262 = Release Notifier(notifier=w32) -> ()  [unwired: 2 in, 3 out]
  n263 = Release Queue(queue=w51, error in (no error)=w50) -> ()  [unwired: 1 in, 3 out]
  n264 = Release Queue(queue=w55, error in (no error)=w54) -> ()  [unwired: 1 in, 3 out]
  n265 = call-poly <vilib>:"Close Input Device.vi"("device ID"=w57) -> ()  [unwired: 9 in, 1 out]
